vi "PositionToReceivePass3rdEnemySide.vi"(6 "y ball":dbl, 8 "error in (no error)":errorcluster, 9 "Robot":refnum<class "Robot.lvclass">, 10 "Game":refnum<class "Game.lvclass">, 11 "PositionToReceivePassSkill in":refnum<class "PositionToReceivePassSkill.lvclass">) -> (0 "error out":errorcluster, 2 "3rdStrikerPosition":dbl[](array[numeric]), 3 "PositionToReceivePassSkill out":refnum<class "PositionToReceivePassSkill.lvclass">)   [LabVIEW 2020, in "PositionToReceivePassSkill.lvclass"]
uses:
  PositionToReceivePassSkill.lvclass
  Game_class/Game.lvclass
  Robot_class/Robot.lvclass
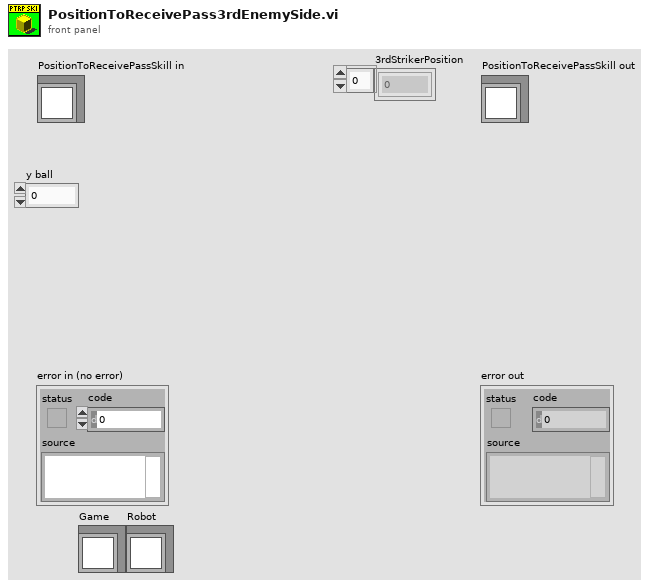
[diagram p1: front panel]
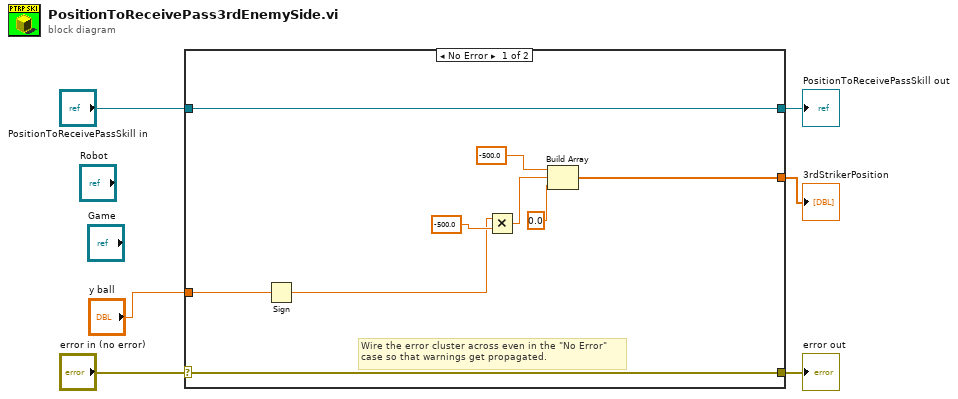
[diagram p0: block diagram]
diagram:
  n1 = case shown="No Error" "error in (no error)" {
    selector: "error in (no error)" -> [w14 w17]
    tunnel: [w14 w17] -> w5
    tunnel: [w15 w16] -> w3
    tunnel: "PositionToReceivePassSkill in" -> [w15 w16]
    tunnel: [w13 _] -> w2
    tunnel: "y ball" -> [w10 _]
    frame No Error {
      # "Wire the error cluster across even in the \"No Error\"\ncase so that warnings get propagated."
      n2 = Sign(1:w10) -> (0:w7:dbl)
      n3 = Multiply(x=w7, y=-500.0 ("element")) -> (x*y=w9:dbl)
      n4 = Build Array(-500.0 ("element"), w9, 0.0 ("element")) -> (w13:dbl[])
    }
    frame Error {
    }
  }
  "error out" <- w5
  "PositionToReceivePassSkill out" <- w3
  "3rdStrikerPosition" <- w2
